vi "Control - Industrial Control.vi"() -> ()   [LabVIEW 2019, in "Control Workspace Object.lvlib"]
doc: "Sample numeric display item."
uses:
  Control Workspace Object.lvlib
  <vilib>/NI VeriStand/Display Template Support/DisplayTemplateSupport.llb/cluster_Screen Item Settings.ctl
  <vilib>/NI VeriStand/Display Template Support/DisplayTemplateSupport.llb/cluster_Graph Scale Settings.ctl
  <vilib>/NI VeriStand/Display Template Support/DisplayTemplateSupport.llb/cluster_Graph Plot Settings.ctl
  NationalInstruments.VeriStand.SystemStorage
  Types/Workspace Object State Variables.ctl
  Types/UI.Refs.ctl
  Types/UDP Streaming Command Cluster.ctl
  Types/UDP Streaming State.ctl
  <vilib>/NI VeriStand/Display Template Support/DisplayTemplateSupport.llb/enum_Display Template Handler Minimal To Workspace.ctl
  Types/Workspace Object Cached Settings.ctl
  <vilib>/NI VeriStand/Execution/Workspace/WorkspaceAPI.ctl
  <vilib>/NI VeriStand/Display Template Support/DisplayTemplateSupport.llb/enum_Display Template Handler Minimal To Widget Msg.ctl
  <vilib>/NI VeriStand/Execution/Workspace/SystemStateRegEventRef.ctl
  <vilib>/NI VeriStand/Execution/Workspace/Target State Info.ctl
  <vilib>/NI VeriStand/Execution/Workspace/Target State.ctl
  <vilib>/NI VeriStand/Execution/Workspace/SystemStateEventRef.ctl
  Shared/Constants.vi
  <vilib>/NI VeriStand/Execution/Workspace/NI VeriStand - Get Multiple Channel Values.vi
  <vilib>/NI VeriStand/Execution/Workspace/NI VeriStand - Set Single Channel Value.vi
  <vilib>/NI VeriStand/Display Template Support/DisplayTemplateSupport.llb/sub_Display Template Handler Custom.vi
  Shared/Control Addon Shared.lvlib
  <vilib>/NI VeriStand/Execution/Workspace/NI_VS Workspace ExecutionAPI.lvlib
  Workspace Shared/Control Workspace Shared.lvlib
  NationalInstruments.VeriStand.ClientAPI
panel:
  in  "Manual Value":bool
  in  "Revert":bool
  in  "Apply":bool
  in  "Manual Output":dbl
  in  "Manual Control":bool
  in  "Setpoint":dbl
  in  "NIVS.System Definition Root":refnum<k24>
  in  "NIVS.Gateway IP Address":string
  in  "Hold":bool
  in  "Autoscale Y":bool=TRUE
  in  "Autoscale X":bool=TRUE
  out "Chart":waveform(dbl)[](graph)
  out "Device":string
  in  "Item.Data":T1
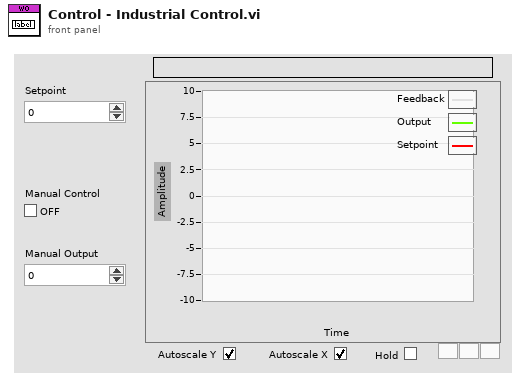
[diagram p1: front panel]
types:
  T1 = typedef "cluster_Screen Item Settings.ctl" = cluster{"Template VI":string, "Position X":i32, "Position Y":i32, "Custom":string, "Show Title Bar":bool, "ID":i32, "Always On Top":bool, "Allow Resize":bool, "Allow Minimize":bool, "Allow Close":bool, "Size to Screen":bool, "Screen.ID":i32, "State":enum16{"Normal", "New"}, "Title":string, "Window Bounds":cluster{"[0]":i16, "[1]":i16, "[2]":i16, "[3]":i16}, "Channel Ref":u64, "Unit":string, "Default Units?":bool, "Flash Limit?":bool, "Color 1":u32, "Color 2":u32, "Color 3":u32, "Color 4":u32, "Bck Color":u32, "Fore Color":u32, "Limit 1":dbl, "Limit 2":dbl, "Limit 3":dbl, "Limit 4":dbl, "Limit Mode 1":i32, "Limit Mode 2":i32, "Limit Mode 3":i32, "Limit Mode 4":i32, "Scale Precision":i32, "Scale Min":dbl, "Scale Max":dbl, "Format":i32, "Precision":i32, "Background Type":i32, "IDs":i32[], "Units":string[], "Labels":string[], "Scale Factor":dbl, "Scale Offset":dbl, "YScale Index":u32[], "XScale":T2, "YScales":T2[], "Plots":T3[], "Update Period":dbl, "History Length":dbl, "My.Ref":refnum<vi>, "Is Control?":bool, "Channel Paths":string[], "Custom Data":variant}
  T2 = typedef "cluster_Graph Scale Settings.ctl" = cluster{"Format":u8, "Precision":u8, "Fit":u8, "Label":string, "Use Default Label":bool, "Label Visible":bool, "Min":dbl, "Max":dbl}
  T3 = typedef "cluster_Graph Plot Settings.ctl" = cluster{"Bar Style":u8, "Fill To":i16, "Fill/PtColor":u32, "Line Style":u8, "Line Width":u8, "Color":u32, "Interp":u8, "Point Style":u8}
  T4 = typedef "Control Workspace Object.lvlib/Workspace Object State Variables.ctl" = cluster{"UI.Refs":T5, "Addon.GUID":string, "Addon.Name":string, "Addon.Type":enum16{"PID", "Industrial"}, "Data.UDPEngineQueue":refnum<queue>, "Data.Found?":bool, "Data.UDPChannels":string[], "Data.PreviousValues":dbl[], "Data.SlowChannels":string[], "Data.PendingChange?":bool, "CachedData.UserEvent":refnum<user-event>, "CachedData.Data":T6, "Addon.Connected?":bool, "NIVS.SysDefRoot":refnum<k24>, "NIVS.Workspace":T7, "NIVS.UserEventRefs":cluster{"Event Registration Refnum":refnum<event-registration>, "SystemChangeEventRef":T8}, "NIVS.SystemStateRefs":T9, "NIVS.LaunchRef":refnum<user-event>, "Setpoint Range":cluster{"Min":dbl, "Max":dbl}, "Output Range":cluster{"Min":dbl, "Max":dbl}}
  T5 = typedef "Control Workspace Object.lvlib/UI.Refs.ctl" = cluster{"Chart":refnum<vi>, "Manual Value":refnum<vi>, "Manual Output":refnum<vi>, "Revert":refnum<vi>, "Apply":refnum<vi>, "Setpoint":refnum<vi>, "Autoscale X":refnum<vi>, "Autoscale Y":refnum<vi>, "Hold":refnum<vi>, "Manual Control":refnum<vi>, "Device":refnum<vi>}
  T6 = typedef "Control Workspace Object.lvlib/Workspace Object Cached Settings.ctl" = cluster{"Path":string}
  T7 = typedef "NI_VS Workspace ExecutionAPI.lvlib/WorkspaceAPI.ctl" = refnum<k24>
  T8 = typedef "NI_VS Workspace ExecutionAPI.lvlib/SystemStateRegEventRef.ctl" = refnum<event-registration>
  T9 = typedef "NI_VS Workspace ExecutionAPI.lvlib/SystemStateEventRef.ctl" = cluster{"CustDatRef":refnum<user-event>, "EvtRef":refnum<k27>, "Target State User Event":refnum<user-event>}
  T10 = typedef "enum_Display Template Handler Minimal To Workspace.ctl" = cluster{"Operation":enum16{"SetCustomData", "DeleteItem"}, "Data":variant}
  T11 = typedef "enum_Display Template Handler Minimal To Widget Msg.ctl" = enum16{"Stop", "LaunchConfigDialog"}
  T12 = typedef "Control Workspace Object.lvlib/UDP Streaming Command Cluster.ctl" = cluster{"Action":T13, "Channels":string[]}
  T13 = typedef "Control Workspace Object.lvlib/UDP Streaming State.ctl" = enum8{"Idle", "Start Acq", "Run", "Stop Acq", "Exit"}
  T14 = cluster{"Event Registration Refnum":refnum<event-registration>, "SystemChangeEventRef":T8}
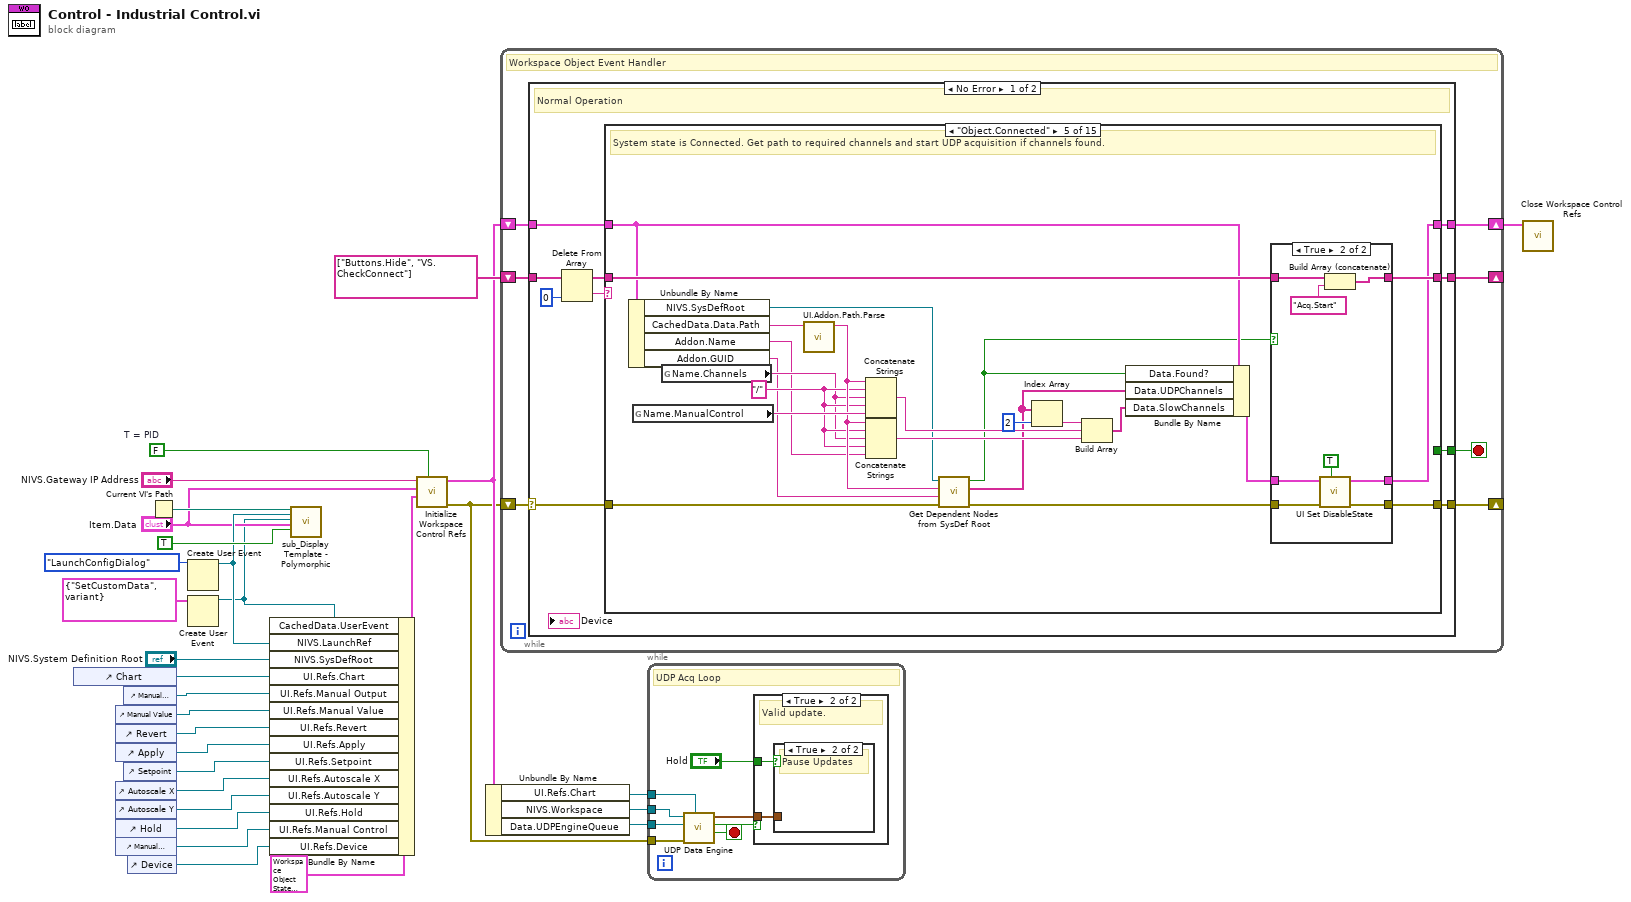
[diagram p0: block diagram]
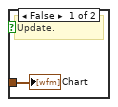
[diagram p3: hidden frame]
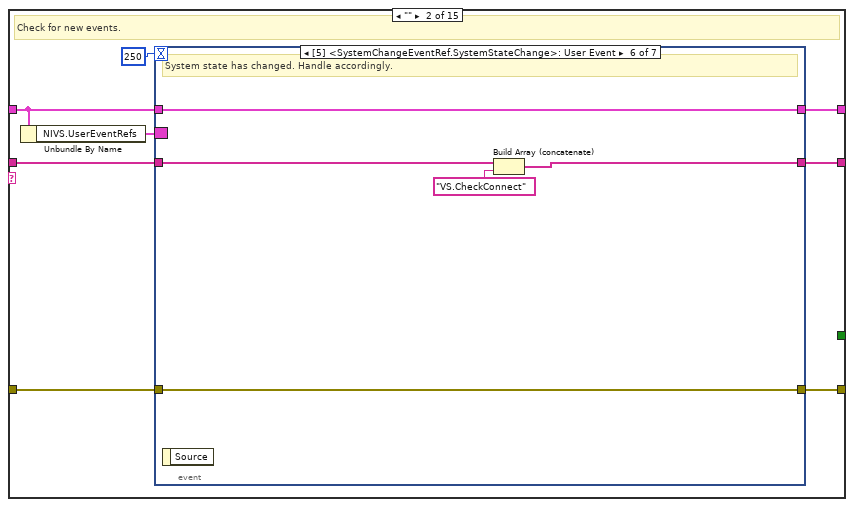
[diagram p5: hidden frame]
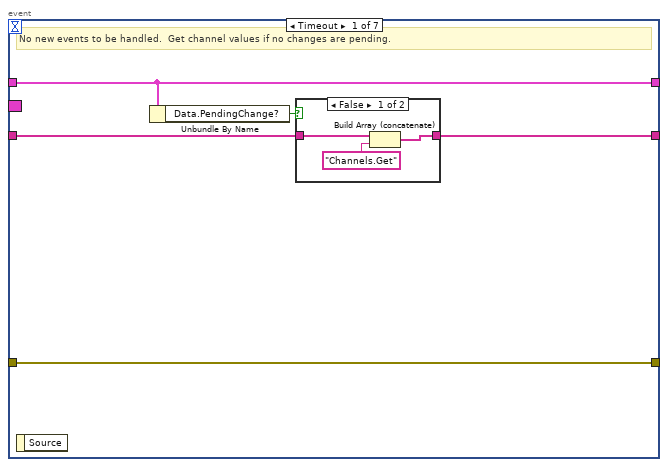
[diagram p6: hidden frame]
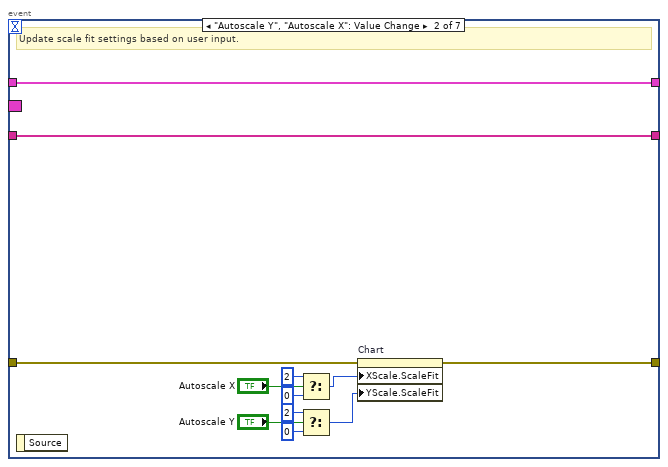
[diagram p8: hidden frame]
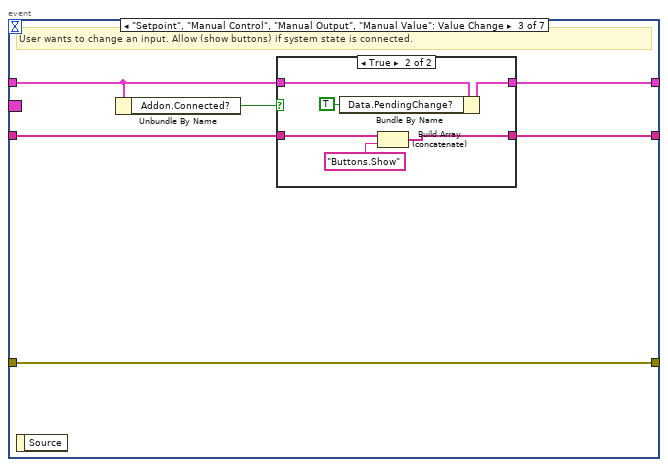
[diagram p9: hidden frame]
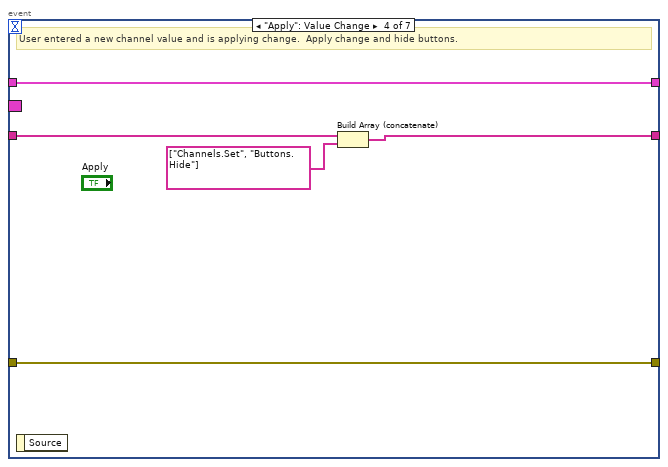
[diagram p11: hidden frame]
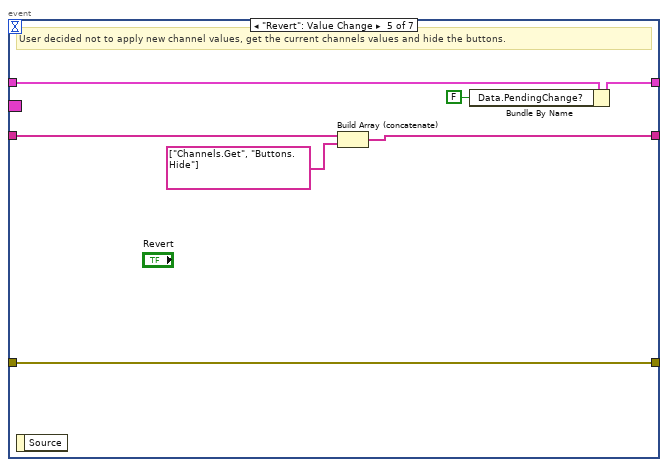
[diagram p12: hidden frame]
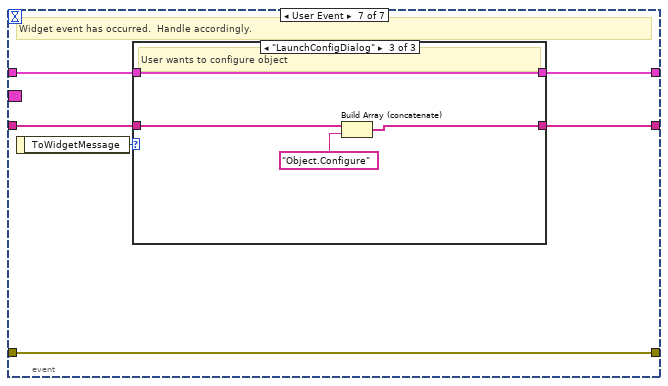
[diagram p13: hidden frame]
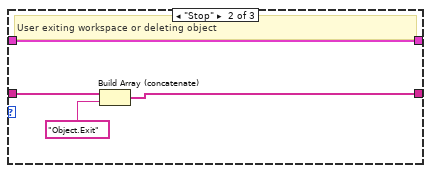
[diagram p15: hidden frame]
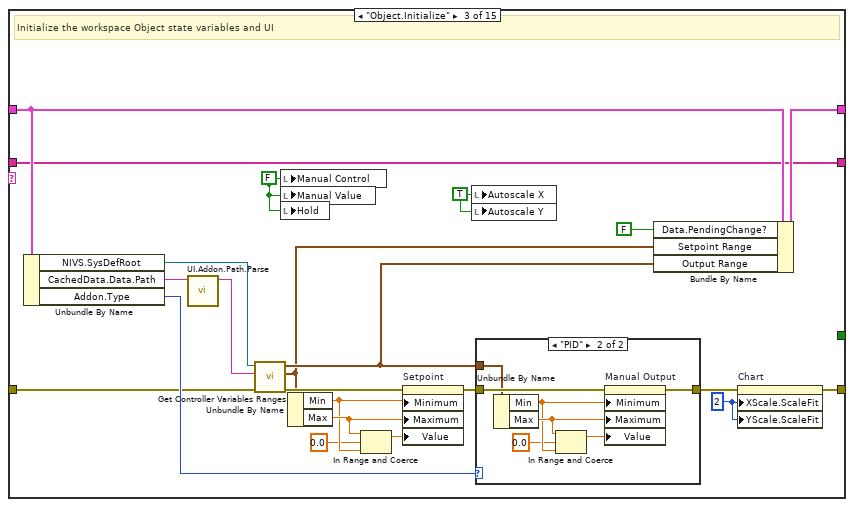
[diagram p16: hidden frame]
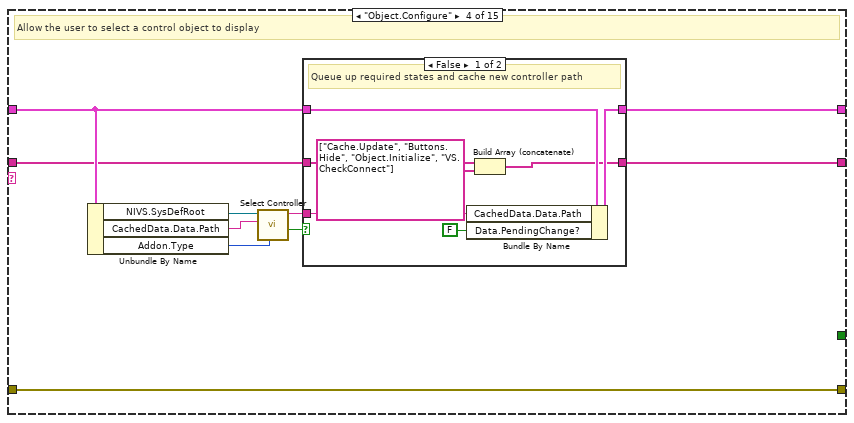
[diagram p18: hidden frame]
diagram:
  w13 = FALSE  # T = PID
  n1 = control-ref of="Chart"() -> (w19:refnum<vi>)
  n2 = control-ref of="Manual Value"() -> (w17:refnum<vi>)
  n3 = control-ref of="Revert"() -> (w16:refnum<vi>)
  n4 = control-ref of="Apply"() -> (w15:refnum<vi>)
  n5 = control-ref of="Autoscale X"() -> (w4:refnum<vi>)
  n6 = control-ref of="Autoscale Y"() -> (w5:refnum<vi>)
  n7 = control-ref of="Hold"() -> (w6:refnum<vi>)
  n8 = control-ref of="Manual Control"() -> (w3:refnum<vi>)
  n9 = control-ref of="Manual Output"() -> (w18:refnum<vi>)
  n10 = control-ref of="Setpoint"() -> (w7:refnum<vi>)
  n11 = control-ref of="Device"() -> (w2:refnum<vi>)
  n12 = Current VI's Path() -> (path=w28:path)
  n13 = Create User Event(user event datatype=enum_Display_Template_Handler_Minimal_To_Widget_Msg."LaunchConfigDialog" ("ToWidgetMessage")) -> (user event=w14:refnum<user-event>)  [unwired: 1 in, 1 out]
  n14 = Create User Event(user event datatype=T10 {"Operation"=enum."SetCustomData", "Data"=variant} ("Data")) -> (user event=w9:refnum<user-event>)  [unwired: 1 in, 1 out]
  n15 = Bundle By Name(cluster=T4 {"UI.Refs"={"Chart"=refnum, "Manual Value"=refnum, "Manual Output"=refnum, "Revert"=refnum, "Apply"=refnum, "Setpoint"=refnum, "Autoscale X"=refnum, "Autoscale Y"=refnum, "Hold"=refnum, "Manual Control"=refnum, "Device"=refnum}, "Addon.GUID"="", "Addon.Name"="", "Addon.Type"=enum."PID", "Data.UDPEngineQueue"=refnum, "Data.Found?"=FALSE, "Data.UDPChannels"=[], "Data.PreviousValues"=[], "Data.SlowChannels"=[], "Data.PendingChange?"=FALSE, "CachedData.UserEvent"=refnum, "CachedData.Data"={"Path"=""}, "Addon.Connected?"=FALSE, "NIVS.SysDefRoot"=refnum, "NIVS.Workspace"=refnum, "NIVS.UserEventRefs"={"Event Registration Refnum"=refnum, "SystemChangeEventRef"=refnum}, "NIVS.SystemStateRefs"={"CustDatRef"=refnum, "EvtRef"=refnum, "Target State User Event"=refnum}, "NIVS.LaunchRef"=refnum, "Setpoint Range"={"Min"=0.0, "Max"=0.0}, "Output Range"={"Min"=0.0, "Max"=0.0}}, "CachedData.UserEvent"=w9, "NIVS.LaunchRef"=w14, "NIVS.SysDefRoot"="NIVS.System Definition Root", "UI.Refs.Chart"=w19, "UI.Refs.Manual Output"=w18, "UI.Refs.Manual Value"=w17, "UI.Refs.Revert"=w16, "UI.Refs.Apply"=w15, "UI.Refs.Setpoint"=w7, "UI.Refs.Autoscale X"=w4, "UI.Refs.Autoscale Y"=w5, "UI.Refs.Hold"=w6, "UI.Refs.Manual Control"=w3, "UI.Refs.Device"=w2) -> (w11:T4)
  n16 = call-poly <vilib>:"sub_Display Template - Polymorphic.vi"("Parent.Path"=w28, "ToWidgetEvent"=w14, "ToWorkspace"=w9, "Item.Data"="Item.Data", "Resizable"=TRUE) -> ()  [unwired: 1 in, 14 out]
  n17 = call "Initialize Workspace Control Refs.vi"("T = PID"=w13, "State Variables in"=w11, "Item.Data"="Item.Data", "NIVS.Gateway IP Address"="NIVS.Gateway IP Address") -> ("error out"=w8:errorcluster, "State Variables out"=w22:T4)  [unwired: 6 in]
  n18 = Unbundle By Name(w22) -> ("UI.Refs.Chart"=w24:refnum<vi>, "NIVS.Workspace"=w23:T7, "Data.UDPEngineQueue"=w21:refnum<queue>)
  n19 = while {
    shift-right: [w35] -> _
    shift-left: string[] ["Buttons.Hide", "VS.CheckConnect"] -> [w36]
    shift-right: [w33] -> w1
    shift-left: w22 -> [w32]
    shift-right: [w34] -> _
    shift-left: w8 -> [w31]
    stop <- w37 stop-if-true
    # "Workspace Object Event Handler"
    n20 = case shown="No Error" w31 {
      selector: w31 -> [w38 w382]
      tunnel: [w47 _] -> w37
      tunnel: w36 -> [w45 w390]
      tunnel: [w42 w390] -> w35
      tunnel: [w41 w387] -> w34
      tunnel: [w40 w389] -> w33
      tunnel: w32 -> [w39 w389]
      frame No Error {
        # "Normal Operation"
        n21 = Delete From Array(array=w45, index=0) -> (deleted portion=w44:string, array with subset deleted=w43:string[])  [unwired: 1 in]
        n22 = case shown="\"Object.Connected\"" w44 {
          tunnel: [_ _ _ _ _ _ _ TRUE _ _ _ _ _ _ _] -> w47
          tunnel: [w50 w57 w137 w160 w189 w215 w219 w245 w252 w260 w261 w272 w278 w293 w353] -> w42
          tunnel: w38 -> [w49 w55 w136 w166 w182 w210 w228 w240 w251 w255 w266 w268 w274 w290 w341]
          tunnel: w43 -> [w50 w56 w137 w159 w198 w215 w220 w245 w252 w260 w261 w272 w278 w293 w353]
          tunnel: w39 -> [w48 w51 w145 w164 w197 w212 w217 w237 w248 w259 w263 w271 w277 w283 w339]
          tunnel: [w49 w54 w144 w166 w177 w211 w229 w239 w251 w254 w265 w267 w273 w289 w340] -> w41
          tunnel: [w48 w53 w148 w163 w179 w213 w218 w237 w248 w259 w263 w271 w277 w288 w338] -> w40
          frame Default {
            # "Do nothing."
          }
          frame "" {
            # "Check for new events."
            n23 = Unbundle By Name(w51) -> ("NIVS.UserEventRefs"=w52:T14)
            n24 = event shown="[5] <SystemChangeEventRef.SystemStateChange>: User Event" {
              selector: w52 -> [_ _ _ _ _ _ _]
              dyn-events: _ -> [_ _ _ _ _ _ _]
              timeout: 250 -> [_ _ _ _ _ _ _]
              tunnel: [w61 w79 w82 w94 w102 w109 w115] -> w57
              tunnel: w56 -> [w62 w79 w83 w95 w103 w110 w114]
              tunnel: w55 -> [w63 w73 w85 w98 w105 w106 w113]
              tunnel: [w63 w72 w85 w98 w105 w106 w113] -> w54
              tunnel: [w60 w78 w84 w97 w100 w107 w111] -> w53
              tunnel: w51 -> [w60 w78 w81 w97 w101 w107 w112]
              event Timeout {
                # "No new events to be handled.  Get channel values if no changes are pending."
                n25 = event-data() -> ()  [unwired: 2 out]
                n26 = Unbundle By Name(w60) -> ("Data.PendingChange?"=w59:bool)
                n27 = case shown="False" w59 {
                  tunnel: w62 -> [w65 w67]
                  tunnel: [w64 w67] -> w61
                  frame False {
                    n28 = Build Array (concatenate)(w65, "Channels.Get") -> (w64:string[])
                  }
                  frame True {
                  }
                }
              }
              event "Autoscale Y", "Autoscale X": Value Change {
                # "Update scale fit settings based on user input."
                n29 = event-data() -> ()  [unwired: 2 out]
                n30 = Select(t=u8 2, s="Autoscale X", f=u8 0 ("X Scale.Scale Fit")) -> (s? t:f=w75:u8)
                n31 = Select(t=u8 2, s="Autoscale Y", f=u8 0 ("X Scale.Scale Fit")) -> (s? t:f=w68:u8)
                n32 = property on="Chart" class="WFChart (strict)"(error in=w73, "XScale.ScaleFit"=w75, "YScale.ScaleFit"=w68) -> (error out=w72:errorcluster)  [unwired: 1 in, 1 out]
              }
              event "Setpoint", "Manual Control", "Manual Output", "Manual Value": Value Change {
                # "User wants to change an input. Allow (show buttons) if system state is connected."
                n33 = event-data() -> ()  [unwired: 2 out]
                n34 = Unbundle By Name(w81) -> ("Addon.Connected?"=w80:bool)
                n35 = case shown="True" w80 {
                  tunnel: w81 -> [w86 w92]
                  tunnel: [w86 w91] -> w84
                  tunnel: w83 -> [w87 w90]
                  tunnel: [w87 w88] -> w82
                  frame False {
                  }
                  frame True {
                    n36 = Bundle By Name(cluster=w92, "Data.PendingChange?"=TRUE ("Pending Change?")) -> (w91:T4)
                    n37 = Build Array (concatenate)(w90, "Buttons.Show") -> (w88:string[])
                  }
                }
              }
              event "Apply": Value Change {
                # "User entered a new channel value and is applying change.  Apply change and hide buttons."
                n38 = event-data() -> ()  [unwired: 2 out]
                n39 = Build Array (concatenate)(w95, string[] ["Channels.Set", "Buttons.Hide"]) -> (w94:string[])
              }
              event "Revert": Value Change {
                # "User decided not to apply new channel values, get the current channels values and hide the buttons."
                n40 = event-data() -> ()  [unwired: 2 out]
                n41 = Build Array (concatenate)(w103, string[] ["Channels.Get", "Buttons.Hide"]) -> (w102:string[])
                n42 = Bundle By Name(cluster=w101, "Data.PendingChange?"=FALSE ("Pending Change?")) -> (w100:T4)
              }
              event User Event {
                # "System state has changed. Handle accordingly."
                n43 = event-data() -> ()  [unwired: 2 out]
                n44 = Build Array (concatenate)(w110, "VS.CheckConnect") -> (w109:string[])
              }
              event User Event {
                # "Widget event has occurred.  Handle accordingly."
                n45 = event-data() -> ("ToWidgetMessage"=w116:T11)  [unwired: 1 out]
                n46 = case shown="\"LaunchConfigDialog\"" w116 {
                  tunnel: [w118 w121 w125] -> w115
                  tunnel: w114 -> [w118 w122 w126]
                  tunnel: w112 -> [w117 w119 w123]
                  tunnel: [w117 w119 w123] -> w111
                  frame Default {
                    # "Do nothing."
                  }
                  frame "Stop" {
                    # "User exiting workspace or deleting object"
                    n47 = Build Array (concatenate)(w122, "Object.Exit") -> (w121:string[])
                  }
                  frame "LaunchConfigDialog" {
                    # "User wants to configure object"
                    n48 = Build Array (concatenate)(w126, "Object.Configure") -> (w125:string[])
                  }
                }
              }
            }
          }
          frame "Object.Initialize" {
            w131 = TRUE ("Manual Control")
            w132 = FALSE ("Manual Control")
            w147 = u8 2 ("X Scale.Scale Fit")
            # "Initialize the workspace Object state variables and UI"
            n49 = Unbundle By Name(w145) -> ("NIVS.SysDefRoot"=w133:refnum<k24>, "CachedData.Data.Path"=w135:string, "Addon.Type"=w140:enum16{"PID", "Industrial"})
            n50 = call "UI.Addon.Path.Parse.vi"("Cached Addon Path"=w135) -> ("Addon Path"=w134:string)  [unwired: 6 in, 4 out]
            n51 = call "Get Controller Variables Ranges.vi"("error in (no error)"=w136, "Path"=w134, "NIVS.SysDef Ref"=w133) -> ("error out"=w143:errorcluster, "Setpoint Range"=w138:cluster{"Min":dbl, "Max":dbl}, "Output Range"=w139:cluster{"Min":dbl, "Max":dbl})  [unwired: 6 in]
            n52 = local write "Manual Control"(w132) -> ()
            n53 = local write "Manual Value"(w132) -> ()
            n54 = local write "Hold"(w132) -> ()
            n55 = Unbundle By Name(w138) -> ("Min"=w129:dbl, "Max"=w130:dbl)
            n56 = In Range and Coerce(upper limit=w130, x=0.0, lower limit=w129) -> (coerced(x)=w128:dbl)  [unwired: 1 out]
            n57 = property on="Setpoint" class="DigNum (strict)"(error in=w143, "Minimum"=w129, "Maximum"=w130, "Value"=w128) -> (error out=w142:errorcluster)  [unwired: 1 in, 1 out]
            n58 = local write "Autoscale X"(w131) -> ()
            n59 = local write "Autoscale Y"(w131) -> ()
            n60 = case shown="\"PID\"" w140 {
              tunnel: w142 -> [w149 w156]
              tunnel: [w149 w155] -> w141
              tunnel: w139 -> [_ w154]
              frame Default {
              }
              frame "PID" {
                n61 = Unbundle By Name(w154) -> ("Min"=w152:dbl, "Max"=w153:dbl)
                n62 = In Range and Coerce(upper limit=w153, x=0.0, lower limit=w152) -> (coerced(x)=w150:dbl)  [unwired: 1 out]
                n63 = property on="Manual Output" class="DigNum (strict)"(error in=w156, "Minimum"=w152, "Maximum"=w153, "Value"=w150) -> (error out=w155:errorcluster)  [unwired: 1 in, 1 out]
              }
            }
            n64 = Bundle By Name(cluster=w145, "Data.PendingChange?"=FALSE ("Pending Change?"), "Setpoint Range"=w138, "Output Range"=w139) -> (w148:T4)
            n65 = property on="Chart" class="WFChart (strict)"(error in=w141, "XScale.ScaleFit"=w147, "YScale.ScaleFit"=w147) -> (error out=w144:errorcluster)  [unwired: 1 in, 1 out]
          }
          frame "Object.Configure" {
            # "Allow the user to select a control object to display"
            n66 = Unbundle By Name(w164) -> ("NIVS.SysDefRoot"=w158:refnum<k24>, "CachedData.Data.Path"=w165:string, "Addon.Type"=w157:enum16{"PID", "Industrial"})
            n67 = call "Select Controller.vi"("Type"=w157, "CD Path"=w165, "NIVS.System Definition Root"=w158) -> ("Cancelled?"=w162:bool, "Custom Device Path Out"=w161:string)  [unwired: 6 in, 1 out]
            n68 = case shown="False" w162 {
              tunnel: w164 -> [w173 w174]
              tunnel: [w172 w174] -> w163
              tunnel: w161 -> [w171 _]
              tunnel: [w169 w175] -> w160
              tunnel: w159 -> [w170 w175]
              frame False {
                # "Queue up required states and cache new controller path"
                n69 = Bundle By Name(cluster=w173, "CachedData.Data.Path"=w171, "Data.PendingChange?"=FALSE) -> (w172:T4)
                n70 = Build Array (concatenate)(w170, string[] ["Cache.Update", "Buttons.Hide", "Object.Initialize", "VS.CheckConnect"]) -> (w169:string[])
              }
              frame True {
                # "User canceled"
              }
            }
          }
          frame "Object.Connected" {
            w186 = "/" ("string")
            # "System state is Connected. Get path to required channels and start UDP acquisition if channels found."
            n71 = Unbundle By Name(w197) -> ("NIVS.SysDefRoot"=w183:refnum<k24>, "CachedData.Data.Path"=w196:string, "Addon.Name"=w184:string, "Addon.GUID"=w181:string)
            n72 = global read "Constants.vi" "Name.ManualControl"() -> (w195:string)
            n73 = global read "Constants.vi" "Name.Channels"() -> (w185:string)
            n74 = call "UI.Addon.Path.Parse.vi"("Cached Addon Path"=w196) -> ("Addon Path"=w194:string)  [unwired: 6 in, 4 out]
            n75 = Concatenate Strings(w194, w186, w185, w186, w195) -> (w193:string)
            n76 = Concatenate Strings(w194, w186, w185, w186, w184) -> (w192:string)
            n77 = call "Get Dependent Nodes from SysDef Root.vi"("error in (no error)"=w182, "GUID"=w181, "Path"=w194, "SysDef Ref"=w183) -> ("error out"=w178:errorcluster, "Channels"=w188:string[], "Found"=w176:bool)  [unwired: 5 in]
            n78 = Index Array(array=w188, index=2) -> (element=w190:string)
            n79 = Build Array(w190, w193, w192) -> (w187:string[])
            n80 = Bundle By Name(cluster=w197, "Data.Found?"=w176, "Data.UDPChannels"=w188, "Data.SlowChannels"=w187) -> (w180:T4)
            n81 = case shown="True" w176 {
              tunnel: w198 -> [w199 w209]
              tunnel: [w199 w208] -> w189
              tunnel: w180 -> [w200 w207]
              tunnel: [w200 w206] -> w179
              tunnel: w178 -> [w201 w205]
              tunnel: [w201 w204] -> w177
              frame False {
              }
              frame True {
                n82 = call "UI Set DisableState.vi"("Enable?"=TRUE, "error in (no error)"=w205, "State Variables in"=w207) -> ("error out"=w204:errorcluster, "State Variables out"=w206:T4)  [unwired: 7 in]
                n83 = Build Array (concatenate)(w209, "Acq.Start") -> (w208:string[])
              }
            }
          }
          frame "Object.Disconnected" {
            n84 = call "UI Set DisableState.vi"("Enable?"=FALSE, "error in (no error)"=w210, "State Variables in"=w212) -> ("error out"=w211:errorcluster, "State Variables out"=w213:T4)  [unwired: 7 in]
          }
          frame "VS.CheckConnect" {
            n85 = Unbundle By Name(w217) -> ("UI.Refs.Device"=w227:refnum<vi>, "NIVS.Workspace"=w226:T7, "NIVS.SysDefRoot"=w225:refnum<k24>, "CachedData.Data.Path"=w224:string)
            n86 = Current VI's Menubar() -> (w223:refnum<k9>)
            n87 = call "UI.Connection.State.Get.vi"("Menu Ref"=w223, "Name Ref"=w227, "error in (no error)"=w228, "Addon Path in"=w224, "NIVS.System Definition Root in"=w225, "NIVS.Workspace Ref in"=w226) -> ("error out"=w229:errorcluster, "Addon Connected?"=w216:bool, "NIVS.System Definition Root out"=w221:refnum<k24>, "NIVS.Workspace Ref out"=w222:T7)  [unwired: 2 in]
            n88 = case shown="False" w216 {
              tunnel: w220 -> [w231 w234]
              tunnel: [w232 w235] -> w219
              frame True {
                n89 = Build Array (concatenate)(w231, "Object.Connected") -> (w232:string[])
              }
              frame False {
                n90 = Build Array (concatenate)(w234, "Object.Disconnected") -> (w235:string[])
              }
            }
            n91 = Bundle By Name(cluster=w217, "NIVS.Workspace"=w222, "NIVS.SysDefRoot"=w221, "Addon.Connected?"=w216) -> (w218:T4)
          }
          frame "Object.Exit" {
            # "Stop current loop.  Queue Stop Acq and Exit to UDP loop."
            n92 = Unbundle By Name(w237) -> ("Data.UDPEngineQueue"=w236:refnum<queue>)
            n93 = Enqueue Element(queue=w236, element=T12 {"Action"=enum."Stop Acq", "Channels"=[]}, error in (no error)=w240) -> (queue out=w243:refnum<queue>, error out=w241:errorcluster)  [unwired: 1 in, 1 out]
            n94 = Enqueue Element(queue=w243, element=T12 {"Action"=enum."Exit", "Channels"=[]}, error in (no error)=w241) -> (error out=w239:errorcluster)  [unwired: 1 in, 2 out]
          }
          frame "Cache.Update" {
            # "Cache any data needing to be permenantly stored with the workspace object."
            n95 = Unbundle By Name(w248) -> ("CachedData.UserEvent"=w246:refnum<user-event>, "CachedData.Data"=w247:T6)
            n96 = Bundle By Name(cluster=T10 {"Operation"=enum."SetCustomData", "Data"=variant} ("event data"), "Data"=w247) -> (w249:T10)
            n97 = Generate User Event(user event=w246, event data cluster=w249) -> ()  [unwired: 2 in, 2 out]
          }
          frame "Acq.Start" {
            # "Send a Start Acq command to the UDP Loop.  Include the channels to  monitor."
            n98 = Unbundle By Name(w259) -> ("Data.UDPEngineQueue"=w253:refnum<queue>, "Data.UDPChannels"=w257:string[])
            n99 = Bundle By Name(cluster=T12 {"Action"=enum."Start Acq", "Channels"=[]}, "Channels"=w257) -> (w256:T12)
            n100 = Enqueue Element(queue=w253, element=w256, error in (no error)=w255) -> (error out=w254:errorcluster)  [unwired: 1 in, 2 out]
          }
          frame "Acq.Disconnect" {
            # "Send Stop Acq to the UDP Acq Loop.  Reset the UI."
            n101 = Unbundle By Name(w263) -> ("Data.UDPEngineQueue"=w262:refnum<queue>)
            n102 = Enqueue Element(queue=w262, element=T12 {"Action"=enum."Stop Acq", "Channels"=[]}, error in (no error)=w266) -> (error out=w265:errorcluster)  [unwired: 1 in, 2 out]
          }
          frame "Buttons.Hide" {
            w269 = FALSE ("Hold")
            # "Hide the apply and revert buttons from the user."
            n103 = property on="Apply" class="Bool"(error in=w268, "Visible"=w269) -> (error out=w270:errorcluster)  [unwired: 1 in, 1 out]
            n104 = property on="Revert" class="Bool"(error in=w270, "Visible"=w269) -> (error out=w267:errorcluster)  [unwired: 1 in, 1 out]
          }
          frame "Buttons.Show" {
            w275 = TRUE ("Hold")
            # "Show the apply and revert buttons to the user."
            n105 = property on="Apply" class="Bool"(error in=w274, "Visible"=w275) -> (error out=w276:errorcluster)  [unwired: 1 in, 1 out]
            n106 = property on="Revert" class="Bool"(error in=w276, "Visible"=w275) -> (error out=w273:errorcluster)  [unwired: 1 in, 1 out]
          }
          frame "Channels.Get" {
            # "Get the current slow speed channel values from VeriStand if no pending change, data paths are valid and system state is connected."
            n107 = Unbundle By Name(w283) -> ("Setpoint Range.Max"=w282:dbl, "Setpoint Range.Min"=w281:dbl, "Data.PendingChange?"=w284:bool, "Output Range.Max"=w280:dbl, "Output Range.Min"=w279:dbl, "Addon.Type"=w287:enum16{"PID", "Industrial"}, "Data.Found?"=w291:bool, "Addon.Connected?"=w292:bool, "NIVS.Workspace"=w286:T7, "Data.SlowChannels"=w285:string[])
            n108 = case shown="False" w284 {
              tunnel: w292 -> [w315 _]
              tunnel: w291 -> [w309 _]
              tunnel: w290 -> [w306 w332]
              tunnel: [w305 w332] -> w289
              tunnel: [w304 w333] -> w288
              tunnel: w287 -> [w303 _]
              tunnel: w286 -> [w302 _]
              tunnel: w285 -> [w300 _]
              tunnel: w283 -> [w299 w333]
              tunnel: w282 -> [w297 _]
              tunnel: w281 -> [w296 _]
              tunnel: w280 -> [w295 _]
              tunnel: w279 -> [w294 _]
              frame False {
                # "No pending data change.  Allow for a get."
                n109 = Compound Arithmetic op=AND(w309, w315) -> (w310:bool)
                n110 = case shown="False" w310 {
                  tunnel: w306 -> [w325 w331]
                  tunnel: [w325 w330] -> w305
                  tunnel: w302 -> [w324 w329]
                  tunnel: [w324 w328] -> w301
                  tunnel: w300 -> [_ w327]
                  tunnel: [dbl[] [0.0, 0.0, 0.0] ("Values") w326] -> w314
                  frame False {
                    # "Do Nothing."
                  }
                  frame True {
                    # "Connected & paths valid"
                    n111 = call-poly <vilib>:"NI VeriStand - Get Channel Value.vi"("error in (no error)"=w331, "Channels"=w327, "WorkspaceManager in"=w329) -> ("error out"=w330:errorcluster, "Values"=w326:dbl[], "WorkspaceManager out"=w328:T7)  [unwired: 6 in]
                  }
                }
                n112 = Index Array(array=w314) -> (element #1=w313:dbl, element #2=w308:dbl, element #3=w307:dbl)  [unwired: 3 in]
                n113 = case shown="\"Industrial\"" w303 {
                  tunnel: w307 -> [w317 w322]
                  tunnel: w295 -> [_ w320]
                  tunnel: w294 -> [_ w319]
                  frame "Industrial" {
                    n114 = To Long Integer(number=w317) -> (32bit integer=w318:i32)
                    n115 = Not Equal To 0?(x=w318) -> (x != 0?=w316:bool)
                    n116 = local write "Manual Value"(w316) -> ()
                  }
                  frame "PID" {
                    n117 = In Range and Coerce(upper limit=w320, x=w322, lower limit=w319) -> (coerced(x)=w321:dbl)  [unwired: 1 out]
                    n118 = local write "Manual Output"(w321) -> ()
                  }
                }
                n119 = To Long Integer(number=w308) -> (32bit integer=w312:i32)
                n120 = In Range and Coerce(upper limit=w297, x=w313, lower limit=w296) -> (coerced(x)=w298:dbl)  [unwired: 1 out]
                n121 = Not Equal To 0?(x=w312) -> (x != 0?=w311:bool)
                n122 = local write "Setpoint"(w298) -> ()
                n123 = local write "Manual Control"(w311) -> ()
                n124 = Bundle By Name(cluster=w299, "NIVS.Workspace"=w301, "Data.PreviousValues"=w314) -> (w304:T4)
              }
              frame True {
                # "A change is pending.  Don't get channels as this would overwrite the pending change."
              }
            }
          }
          frame "Channels.Set" {
            # "Set Channels if data paths are valid and system state is connected and there is a change in the data value."
            n125 = Unbundle By Name(w339) -> ("Data.Found?"=w344:bool, "Addon.Connected?"=w347:bool, "Data.PreviousValues"=w346:dbl[], "Data.SlowChannels"=w348:string[], "NIVS.Workspace"=w336:T7, "Addon.Type"=w334:enum16{"PID", "Industrial"})
            n126 = case shown="\"PID\"" w334 {
              tunnel: [w355 "Manual Output"] -> w342
              frame "Industrial" {
                n127 = Boolean To (0,1)(Boolean="Manual Value") -> (0, 1=w355:i16)
              }
              frame "PID" {
              }
            }
            n128 = Boolean To (0,1)(Boolean="Manual Control") -> (0, 1=w343:i16)
            n129 = Build Array("Setpoint", w343, w342) -> (w349:dbl[])
            n130 = Not Equal?(x=w346, y=w349) -> (x != y?=w352:bool[])
            n131 = Compound Arithmetic op=AND(w344, w347) -> (w345:bool)
            n132 = case shown="True" w345 {
              tunnel: w352 -> [_ w365]
              tunnel: w349 -> [_ w364]
              tunnel: w341 -> [w358 w363]
              tunnel: [w358 w362] -> w340
              tunnel: w336 -> [w357 w361]
              tunnel: [w357 w360] -> w335
              tunnel: w348 -> [_ w359]
              frame False {
                # "Do nothing"
              }
              frame True {
                # "Connected & paths valid"
                n133 = for {
                  shift-right: [w371] -> w362
                  shift-left: w363 -> [w372]
                  shift-right: [w370] -> w360
                  shift-left: w361 -> [w369]
                  tunnel: w365 -> [w368] mode=indexing
                  tunnel: w364 -> [w367] mode=indexing
                  tunnel: w359 -> [w366] mode=indexing
                  n134 = case shown="True" w368 {
                    tunnel: w372 -> [w374 w380]
                    tunnel: [w374 w379] -> w371
                    tunnel: [w373 w378] -> w370
                    tunnel: w369 -> [w373 w377]
                    tunnel: w367 -> [_ w376]
                    tunnel: w366 -> [_ w375]
                    frame False {
                      # "Do nothing"
                    }
                    frame True {
                      # "Update channel"
                      n135 = call-poly <vilib>:"NI VeriStand - Set Channel Value.vi"("error in (no error)"=w380, "Value"=w376, "Channel"=w375, "WorkspaceManager in"=w377) -> ("error out"=w379:errorcluster, "WorkspaceManager out"=w378:T7)  [unwired: 6 in]
                    }
                  }
                }
              }
            }
            n136 = Bundle By Name(cluster=w339, "Data.PendingChange?"=FALSE ("Pending Change?"), "NIVS.Workspace"=w335) -> (w338:T4)
          }
        }
      }
      frame Error {
        # "Handle Errors."
        n137 = Unbundle By Name(w382) -> ("code"=w386:i32)
        n138 = Equal?(x=-307654, y=w386) -> (x = y?=w384:bool)
        n139 = Select(t=errorcluster {"status"=FALSE, "code"=0, "source"=""}, s=w384, f=w382) -> (s? t:f=w381:errorcluster)
        n140 = call <vilib>:"Simple Error Handler.vi"("error in (no error)"=w381) -> ("error out"=w388:errorcluster)  [unwired: 4 in, 4 out]
        n141 = call <vilib>:"Clear Errors.vi"("error in (no error)"=w388) -> ("error out"=w387:errorcluster)  [unwired: 5 in, 1 out]
      }
    }
  }
  n142 = while {
    tunnel: w23 -> [w393]
    tunnel: w21 -> [w398]
    tunnel: w24 -> [w394]
    tunnel: w8 -> [w392]
    stop <- w397 stop-if-true
    # "UDP Acq Loop"
    n143 = call "UDP Data Engine.vi"("WaveformChart Ref"=w394, "error in (no error)"=w392, "UDP Engine Queue"=w398, "WorkspaceManager"=w393) -> ("Exit"=w397:bool, "Update?"=w391:bool, "Waveform"=w395:waveform(dbl)[])  [unwired: 4 in, 1 out]
    n144 = case shown="True" w391 {
      tunnel: "Hold" -> [_ w400]
      tunnel: w395 -> [_ w399]
      frame False {
        # "Do Nothing."
      }
      frame True {
        # "Valid update."
        n145 = case shown="True" w400 {
          tunnel: w399 -> [w401 _]
          frame False {
            # "Update."
            "Chart" <- w401
          }
          frame True {
            # "Pause Updates"
          }
        }
      }
    }
  }
  n146 = call "Close Workspace Control Refs.vi"("State Variables in"=w1) -> ()  [unwired: 11 in]
